vi "Initialize.vi"(7 "Limit Name":string="Setpoint.ch%d.SP", 8 "error in":errorcluster, 9 "Number of Channels":u32=1, 10 "Instance Name":string="PluginName", 11 "Humidity Limit in":refnum<class "Humidity Limit.lvclass">) -> (0 "error out":errorcluster caption="error in", 2 "Channel":T1[](array[typedef]), 3 "Humidity Limit out":refnum<class "Humidity Limit.lvclass">)   [LabVIEW 2023, in "Humidity Limit.lvclass"]
uses:
  Humidity Limit.lvclass
  Humidity Limit.lvclass/Humidity Limit.ctl
  Parents/Limit/Limit.lvclass
  Utilities/Channel.ctl
  Utilities/Utilities.lvlib
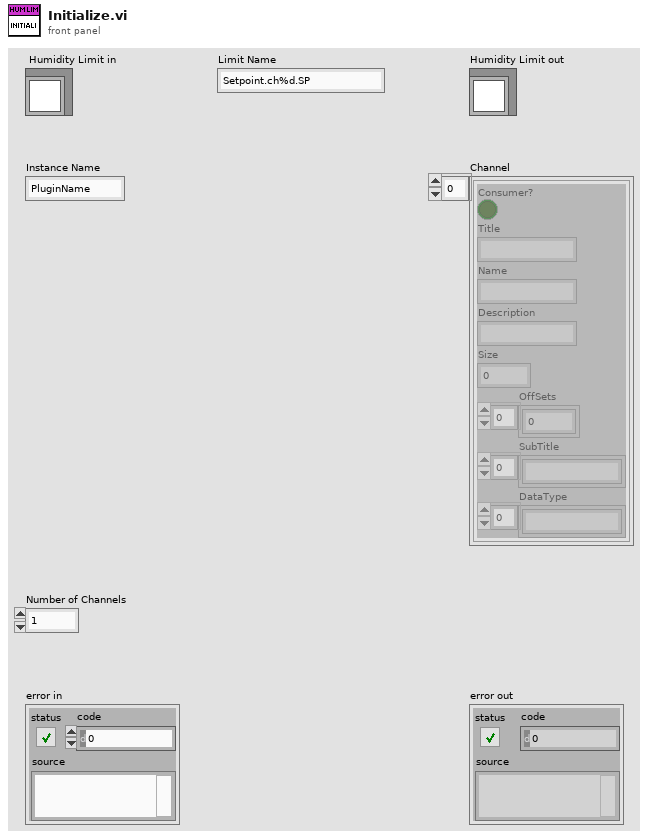
[diagram p1: front panel]
types:
  T1 = typedef "Utilities.lvlib/Channel.ctl" = cluster{"Consumer?":bool, "Title":string, "Name":string, "Description":string, "Size":i32, "OffSets":i32[], "SubTitle":string[], "DataType":string[]}
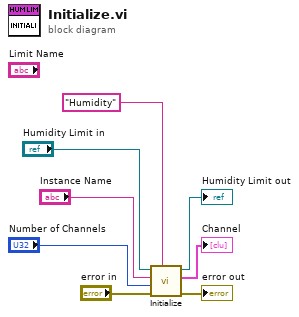
[diagram p0: block diagram]
diagram:
  n1 = call-parent "Initialize.vi"("Limit Name"="Humidity", "error in"="error in", "Number of Channels"="Number of Channels", "Instance Name"="Instance Name", "Limit in"="Humidity Limit in") -> ("error out"=→"error out":errorcluster, "Channel"=→"Channel":T1[], "Limit out"=→"Humidity Limit out":refnum<class "Humidity Limit.lvclass">)  [unwired: 4 in]
